vi "Flatten.vi"(6 "Width Unit (points)":enum16{"Points", "Data"}(ring), 8 "error in (no error)":errorcluster, 9 "width":dbl=3.0 min=3.0, 10 "threshold":dbl format="%0.2f", 11 "XY-data":cluster{"X-array":dbl[], "Y-array":dbl[]}[](array[cluster])) -> (0 "error out":errorcluster, 3 "XY-data out":cluster{"X-array":dbl[], "Y-array":dbl[]}[](array[cluster]) {"Y-array" format="%.2p"; "X-array" format="%.2p"})   [LabVIEW 2019, in "xy_utilities.lvlib"]
doc: "Add <b>x</b> to the x array of <b>XY-data</b>\nAdd <b>y</b> to the y array of <b>XY-data</b>\n\nWire data to the data input to determine the polymorphic instance to use or manually select the instance."
uses:
  xy_utilities.lvlib
  subVIs/Peak Detector (multiple).vi
  subVIs/Subtract float (single).vi
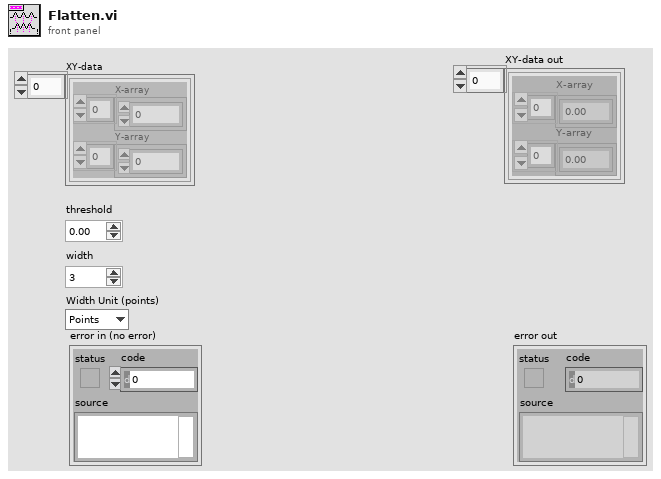
[diagram p1: front panel]
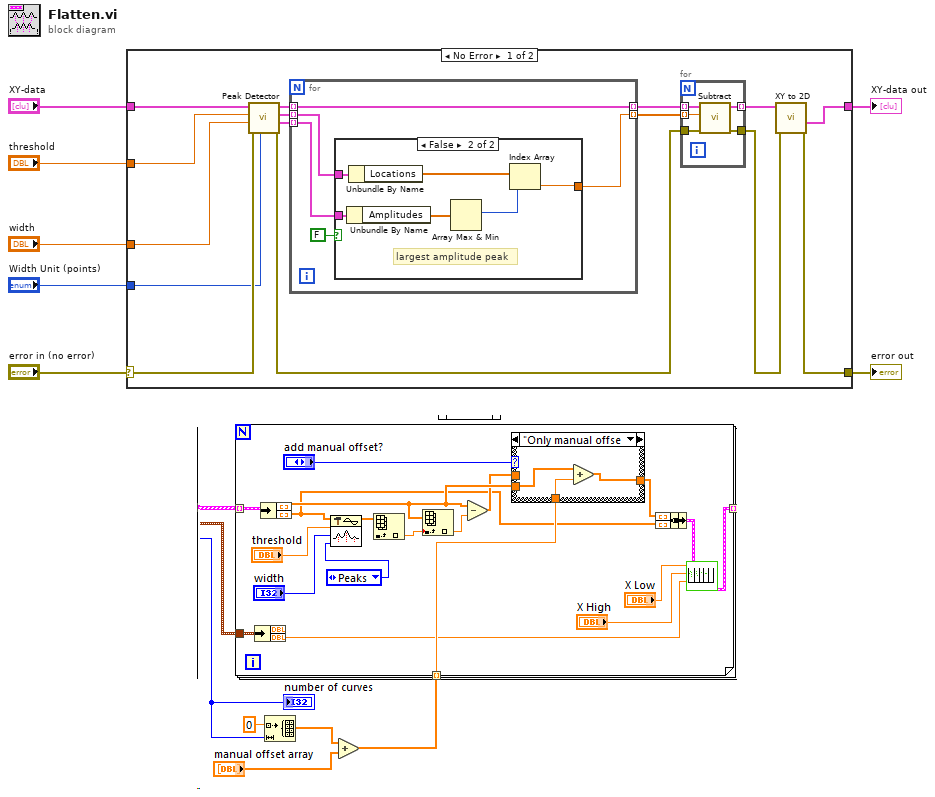
[diagram p0: block diagram]
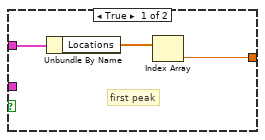
[diagram p2: hidden frame]
diagram:
  n1 = case shown="No Error" "error in (no error)" {
    selector: "error in (no error)" -> [w21 w43]
    tunnel: [w19 w43] -> w6
    tunnel: "XY-data" -> [w22 w42]
    tunnel: [w20 w42] -> w4
    tunnel: "threshold" -> [w18 _]
    tunnel: "width" -> [w17 _]
    tunnel: "Width Unit (points)" -> [w14 _]
    frame No Error {
      n2 = call-poly "Peak Detector.vi"("Width Unit (points)"=w14, "error in (no error)"=w21, "width"=w17, "threshold"=w18, "XY-data"=w22) -> ("error out"=w10:errorcluster, "Amplitudes"=w13:cluster{"Amplitudes":dbl[]}[], "Locations"=w15:cluster{"Locations":dbl[]}[], "XY-data out"=w16:cluster{"X-array":dbl[], "Y-array":dbl[]}[])  [unwired: 3 in]
      n3 = for {
        tunnel: w16 -> [w29] mode=indexing
        tunnel: w15 -> [w32] mode=indexing
        tunnel: [w29] -> w12 mode=indexing
        tunnel: w13 -> [w31] mode=indexing
        tunnel: [w28] -> w11 mode=indexing
        n4 = case shown="False" FALSE {
          tunnel: w32 -> [w35 w41]
          tunnel: [w34 w36] -> w28
          tunnel: w31 -> [_ w40]
          frame True {
            # "first peak"
            n5 = Unbundle By Name(w35) -> ("Locations"=w33:dbl[])
            n6 = Index Array(array=w33) -> (element=w34:dbl)  [unwired: 1 in]
          }
          frame False {
            # "largest amplitude peak"
            n7 = Unbundle By Name(w40) -> ("Amplitudes"=w39:dbl[])
            n8 = Unbundle By Name(w41) -> ("Locations"=w38:dbl[])
            n9 = Array Max & Min(array=w39) -> (max index (indices)=w37:i32)  [unwired: 3 out]
            n10 = Index Array(array=w38, index=w37) -> (element=w36:dbl)
          }
        }
      }
      n11 = for {
        tunnel: w12 -> [w27] mode=indexing
        tunnel: w11 -> [w26] mode=indexing
        tunnel: w10 -> [w25]
        tunnel: [w24] -> w8
        tunnel: [w23] -> w9 mode=indexing
        n12 = call-poly "Subtract.vi"("error in (no error)"=w25, "x (0)"=w26, "XY-data"=w27) -> ("error out"=w24:errorcluster, "XY-data out"=w23:cluster{"X-array":dbl[], "Y-array":dbl[]})  [unwired: 7 in]
      }
      n13 = call "XY to 2D.vi"("error in (no error)"=w8, "XY-data"=w9) -> ("error out"=w19:errorcluster, "Interpolated XY-data out"=w20:cluster{"X-array":dbl[], "Y-array":dbl[]}[])  [unwired: 6 in, 2 out]
    }
    frame Error {
    }
  }
  "error out" <- w6
  "XY-data out" <- w4
